vi "Main.vi"() -> ()   [LabVIEW 2017]
uses:
  type defs/action buttons.ctl
  type defs/mode buttons.ctl
  type defs/state.ctl
  type defs/data.ctl
  <vilib>/vision/Image Controls.llb/IMAQ Image.ctl
  type defs/task.ctl
  <vilib>/myRIO/Instrument Drivers/Onboard IO/DIO/typedefs/DIO Reference.ctl
  <vilib>/myRIO/Common/Instrument Driver Framework/Utilities/typedefs/myRIO Generic Hardware Reference.ctl
  <vilib>/myRIO/Common/Instrument Driver Framework/Utilities/typedefs/Hardware Version Enum.ctl
  <vilib>/myRIO/Common/Instrument Driver Framework/Utilities/typedefs/myRIO v1.0 Reference.ctl
  <vilib>/myRIO/Common/Instrument Driver Framework/Utilities/typedefs/Generic FPGA Reference.ctl
  <vilib>/myRIO/Common/Instrument Driver Framework/myRIO v1.0/DIO/typedefs/DIO Channels List.ctl
  <vilib>/myRIO/Common/Instrument Driver Framework/myRIO v1.0/DIO/typedefs/DIO Channels Enum.ctl
  <vilib>/userdefined/High Color/nirio_resource_hc.ctl
  <vilib>/myRIO/Common/Instrument Driver Framework/Utilities/vis/Is FPGA Ref Available.vi
  <vilib>/myRIO/Common/Instrument Driver Framework/myRIO v1.0/DIO/vis/myRIO v1.1 Open DIO.vi
  <vilib>/myRIO/Instrument Drivers/Onboard IO/DIO/vis/Write.vi
  <vilib>/myRIO/Instrument Drivers/Onboard IO/DIO/vis/Read.vi
  <vilib>/myRIO/Common/Instrument Driver Framework/Utilities/vis/Validate Channels.vi
  <vilib>/myRIO/Common/Instrument Driver Framework/myRIO v1.0/DIO/vis/myRIO v1.0 Reserve DIO.vi
  <vilib>/myRIO/Common/Instrument Driver Framework/myRIO v1.0/UART/vis/myRIO v1.0 Close UART.vi
  <vilib>/myRIO/Common/Instrument Driver Framework/myRIO v1.0/Resource Manager/vis/myRIO v1.0 Reserve Channel List.vi
  <vilib>/myRIO/Common/Instrument Driver Framework/myRIO v1.0/DIO/vis/myRIO v1.0 Build MUX Configuration DIO.vi
  <vilib>/myRIO/Common/Instrument Driver Framework/myRIO v1.0/Resource Manager/vis/myRIO v1.0 Reserve Channel.vi
  <vilib>/myRIO/Common/Instrument Driver Framework/myRIO v1.0/Resource Manager/vis/myRIO v1.0 Unreserve Channel.vi
  <vilib>/myRIO/Common/Instrument Driver Framework/myRIO v1.0/Resource Manager/vis/myRIO v1.0 Create Configuration List.vi
  <vilib>/myRIO/Common/Instrument Driver Framework/myRIO v1.0/Resource Manager/vis/myRIO v1.0 Build Mutex Name.vi
  <vilib>/Utility/VariantDataType/GetNumericInfo.vi
  <vilib>/Utility/error.llb/Error Cluster From Error Code.vi
  <vilib>/myRIO/Common/Instrument Driver Framework/myRIO v1.0/myRIO v1.1 Open.vi
  <vilib>/myRIO/Common/Instrument Driver Framework/Utilities/vis/IO Manager.vi
  <vilib>/myRIO/Common/Instrument Driver Framework/Utilities/vis/Configuration Manager.vi
  <vilib>/myRIO/Common/Instrument Driver Framework/myRIO v1.0/Resource Manager/vis/myRIO v1.0 Configure IO.vi
  <vilib>/myRIO/Common/Instrument Driver Framework/myRIO v1.0/myRIO v1.0 Close.vi
  <vilib>/myRIO/Common/Instrument Driver Framework/myRIO v1.0/DIO/vis/myRIO v1.0 Write DIO.vi
  <vilib>/myRIO/Common/Instrument Driver Framework/myRIO v1.0/DIO/vis/myRIO v1.0 Read DIO.vi
  <vilib>/myRIO/Common/Instrument Driver Framework/Utilities/vis/FPGA Ref Manager.vi
  <vilib>/myRIO/Common/Instrument Driver Framework/myRIO v1.0/myRIO v1.0 Reset FPGA.vi
  <vilib>/myRIO/Common/Instrument Driver Framework/myRIO v1.0/IRQ/vis/myRIO v1.0 IRQ Info FGV.vi
  <vilib>/myRIO/Common/Instrument Driver Framework/myRIO v1.0/IRQ/vis/myRIO v1.0 Timer IRQ Info FGV.vi
  <vilib>/myRIO/Common/Instrument Driver Framework/myRIO v1.0/IRQ/vis/myRIO v1.0 ISR Agent.vi
  <vilib>/myRIO/Express VI/Onboard Devices/LED/LED Express VI.xnode
  <vilib>/myRIO/Instrument Drivers/Onboard IO/DIO/vis/myRIO DIO Open.xnode
  <vilib>/myRIO/Express VI/Onboard Devices/Button/Button Express VI.xnode
  <vilib>/vision/NI_Vision_Development_Module.lvlib
  <vilib>/myRIO/Instrument Drivers/Onboard IO/DIO/DIO.lvlib
  <vilib>/myRIO/Instrument Drivers/Utilities/Utilities.lvlib
panel:
  out "error out":errorcluster
  out "Class (Particle Classification 1)":string
  out "number img":i32
  in  "mode buttons":T1
  out "image display":T2(plugin-control)
  in  "action buttons":T3
  in  "Stop":bool
  # "Machine\nVision\nApp"
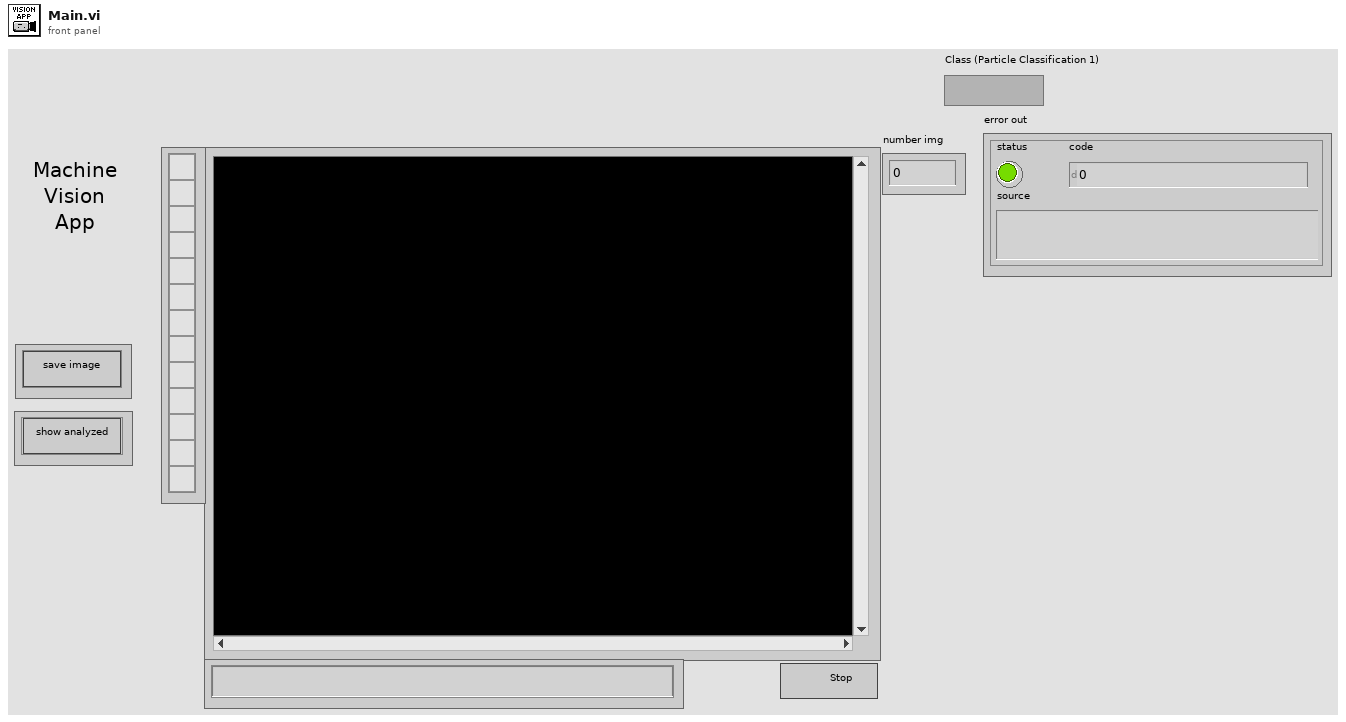
[diagram p1: front panel]
types:
  T1 = typedef "mode buttons.ctl" = cluster{"show analyzed":bool}
  T2 = typedef "IMAQ Image.ctl" = refnum<image>
  T3 = typedef "action buttons.ctl" = cluster{"save image":bool}
  T4 = typedef "data.ctl" = cluster{"save image":bool, "qsm":cluster{"Webcam image ref":T2, "Analyzed image ref":T2, "Stop webcam":bool}, " image ref":T2, "number img":i32}
  T5 = typedef "state.ctl" = enum16{"(qsm) schedule", "(qsm) initialize", "(qsm) release", "(qsm) clean up", "(qsm) shutdown", "(myRIO) initialize", "(myRIO) clean up", "(myRIO) update ports", "(image) get", "(image) analyze", "(image) overlay", "(image) show", "save image", "state A", "state B", "state C", "state D", "state E", "state F", "state G", "state H"}
  T6 = typedef "DIO.lvlib/DIO Reference.ctl" = cluster{"myRIO Reference":T7, "DIO Channels List":T11}
  T7 = typedef "myRIO Generic Hardware Reference.ctl" = cluster{"myRIO Model":T8, "myRIO Hardware Reference":T9}
  T8 = typedef "Hardware Version Enum.ctl" = enum16{"Unknown", "myRIO-1900", "myRIO-1950", "roboRIO", "NI ELVIS RIO CM"}
  T9 = typedef "myRIO v1.0 Reference.ctl" = cluster{"Generic FPGA Reference":T10, "Allow multiple opens":bool}
  T10 = typedef "Generic FPGA Reference.ctl" = refnum<k20>
  T11 = typedef "DIO Channels List.ctl" = T12[]
  T12 = typedef "DIO Channels Enum.ctl" = enum16{"Not Connected", "C/DIO0", "C/DIO1", "C/DIO2", "C/DIO3", "C/DIO4", "C/DIO5", "C/DIO6", "C/DIO7", "A/DIO0", "A/DIO1", "A/DIO2", "A/DIO3", "A/DIO4", "A/DIO5", "A/DIO6", "A/DIO7", "A/DIO8", "A/DIO9", "A/DIO10", "A/DIO11", "A/DIO12", "A/DIO13", "A/DIO14", "A/DIO15", "B/DIO0", "B/DIO1", "B/DIO2", "B/DIO3", "B/DIO4", "B/DIO5", "B/DIO6", "B/DIO7", "B/DIO8", "B/DIO9", "B/DIO10", "B/DIO11", "B/DIO12", "B/DIO13", "B/DIO14", "B/DIO15", "LED0", "LED1", "LED2", "LED3", "Button0", "DIO/DIO0", "DIO/DIO1", "DIO/DIO2", "DIO/DIO3", "DIO/DIO4", "DIO/DIO5", "DIO/DIO6", "DIO/DIO7", "DIO/DIO8", "DIO/DIO9", "SPI/CS0", "SPI/CS1", "SPI/CS2", "SPI/CS3", "LED RADIO (Green)", "LED RADIO (Red)", "LED COMM (Green)", "LED COMM (Red)", "LED MODE (Green)", "LED MODE (Red)"}
  T13 = typedef "nirio_resource_hc.ctl" = tag
  T14 = typedef "task.ctl" = T5[]
  T15 = typedef "Image Type" = u32
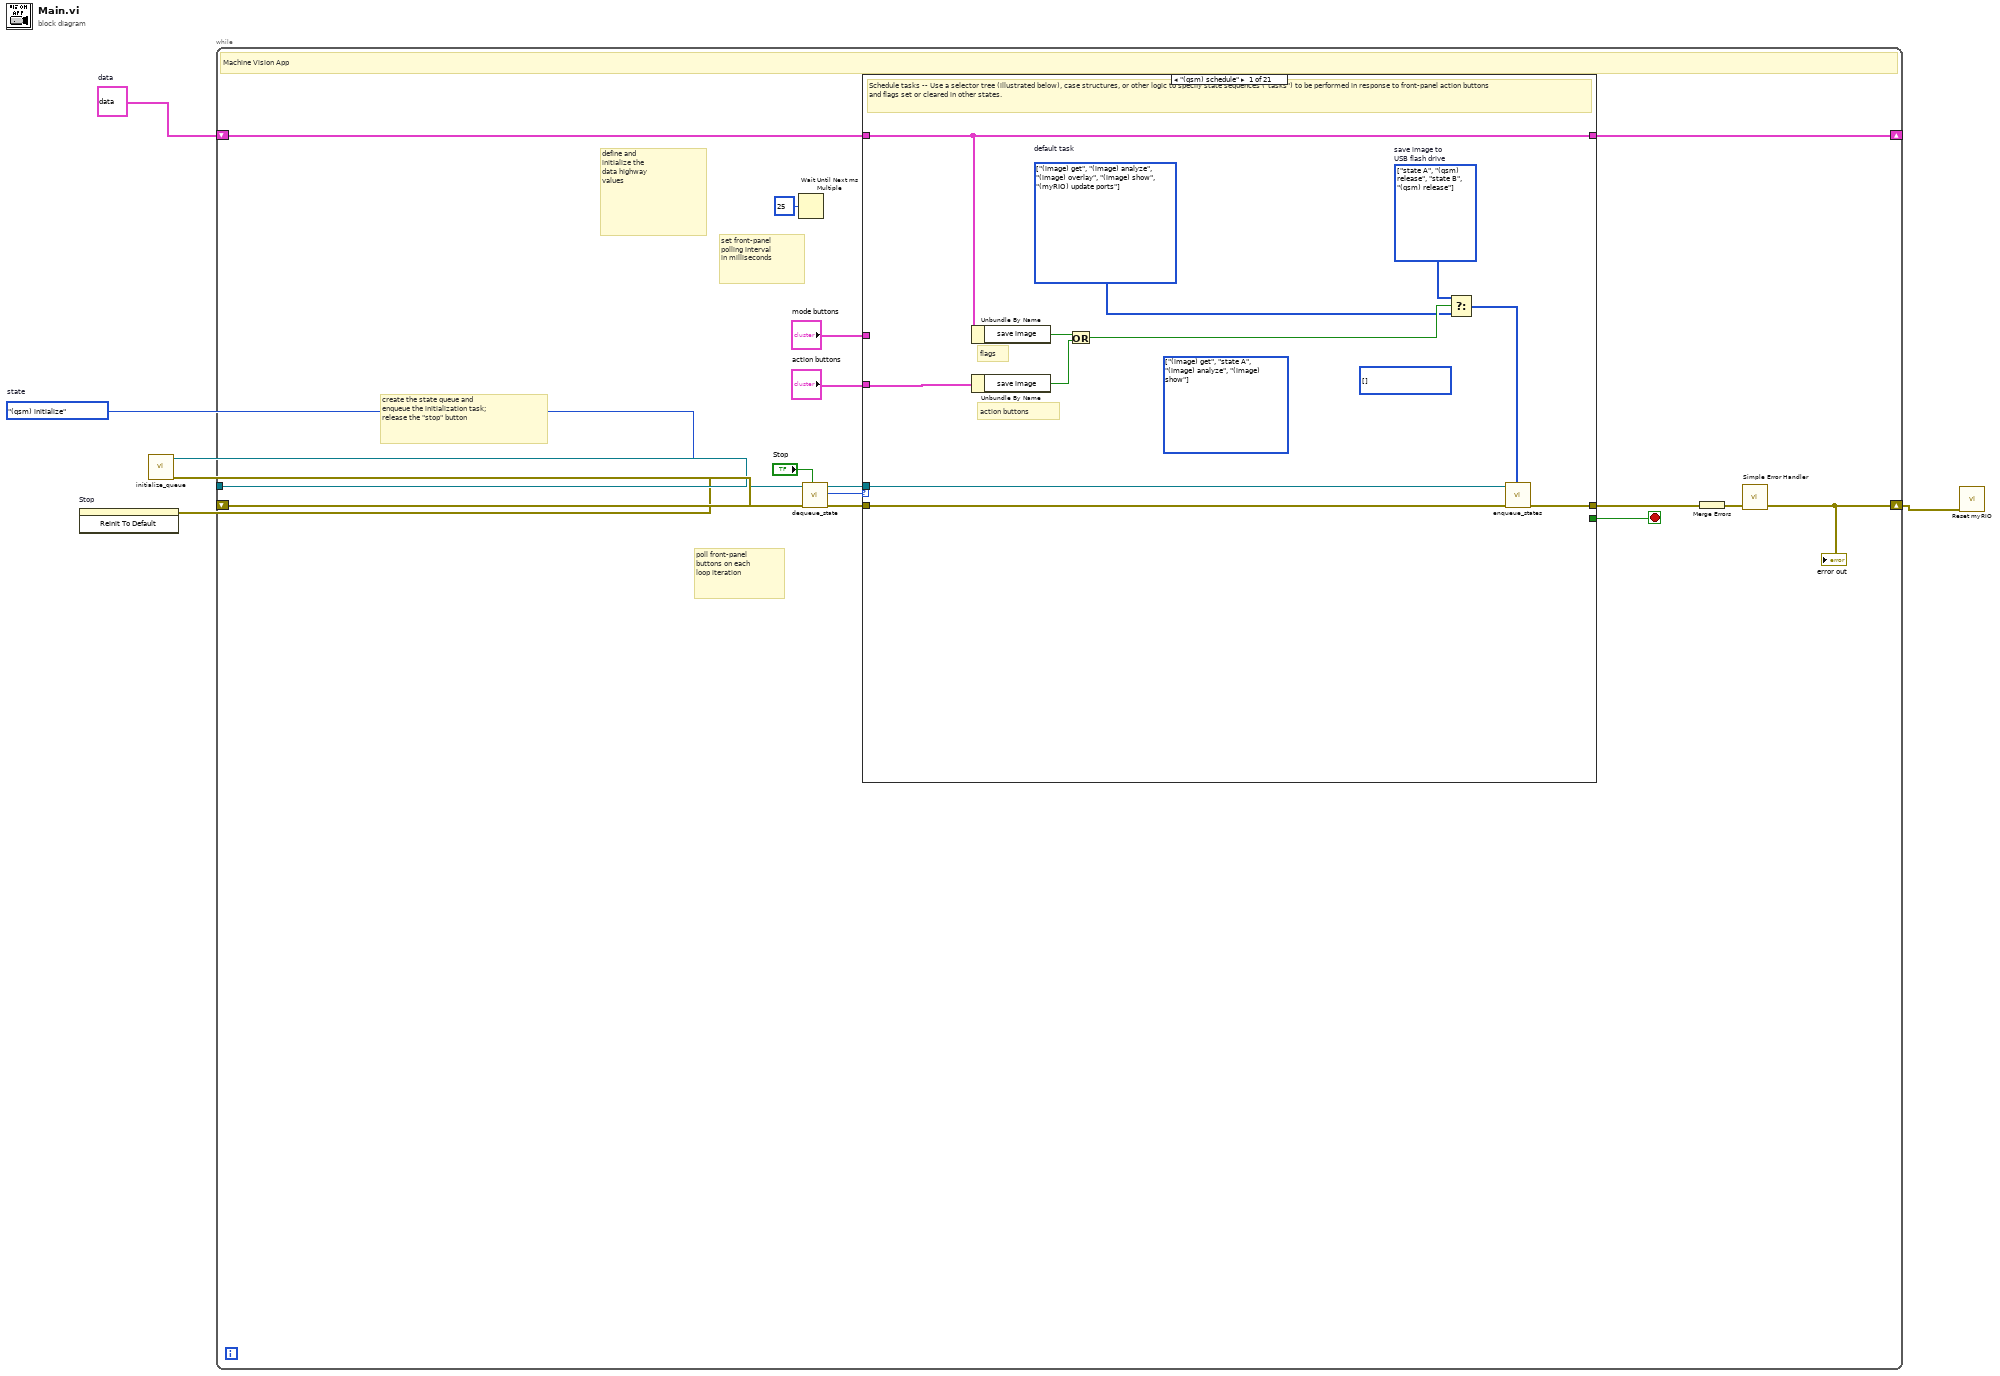
[diagram p0: block diagram]
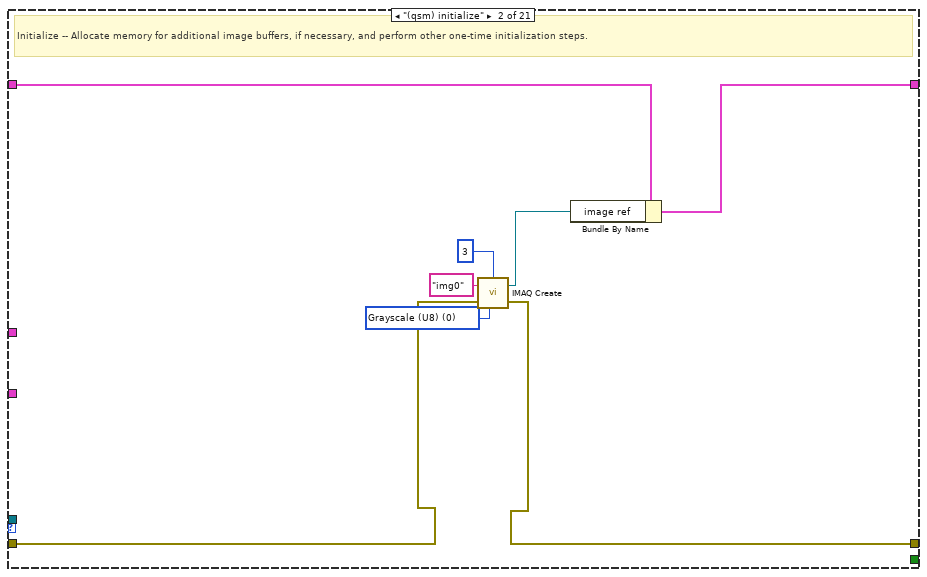
[diagram p2: hidden frame]
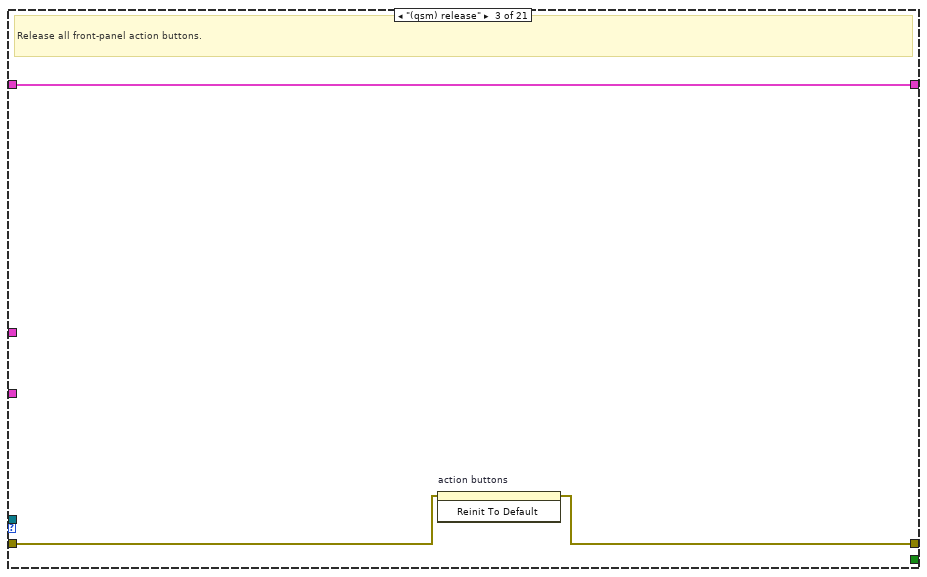
[diagram p3: hidden frame]
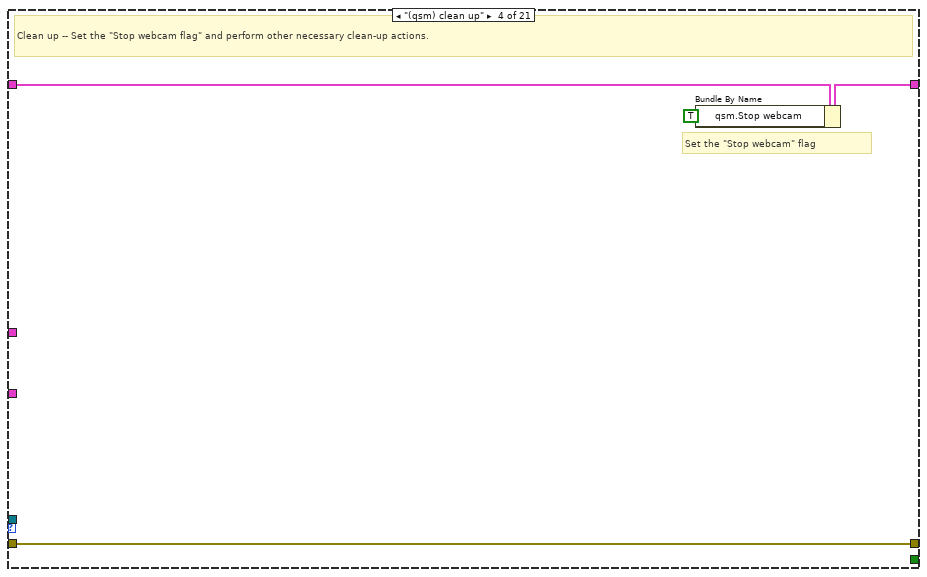
[diagram p4: hidden frame]
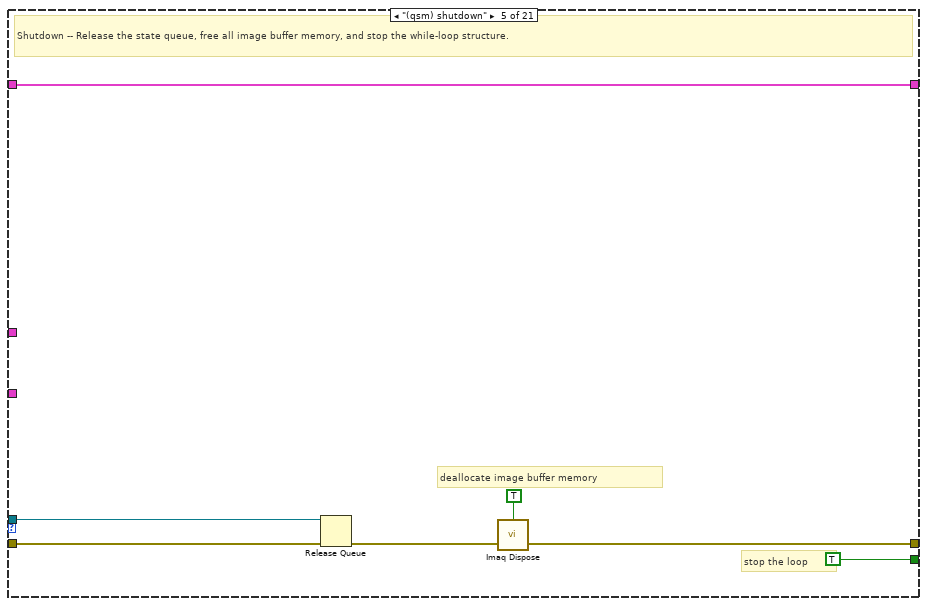
[diagram p5: hidden frame]
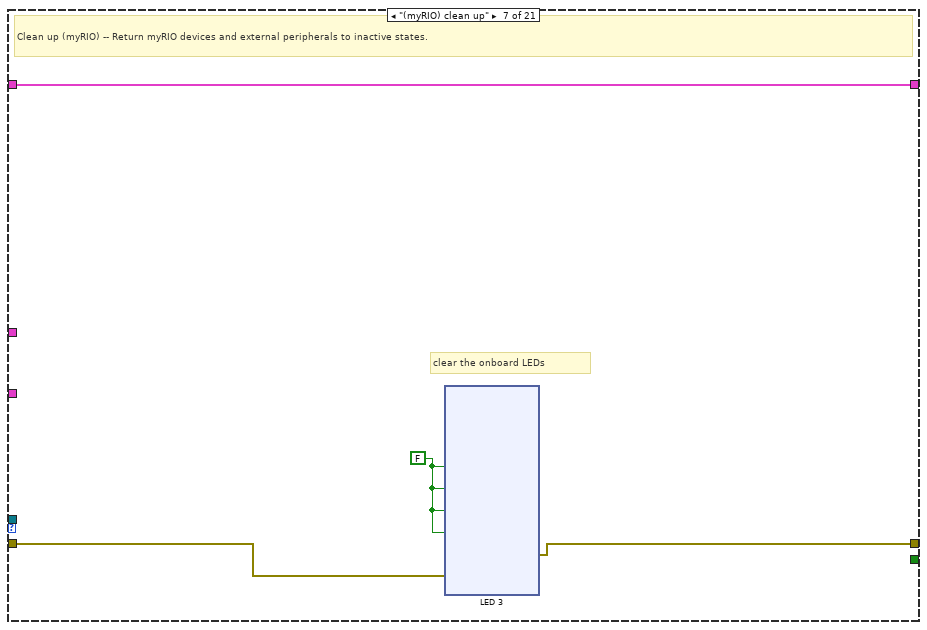
[diagram p7: hidden frame]
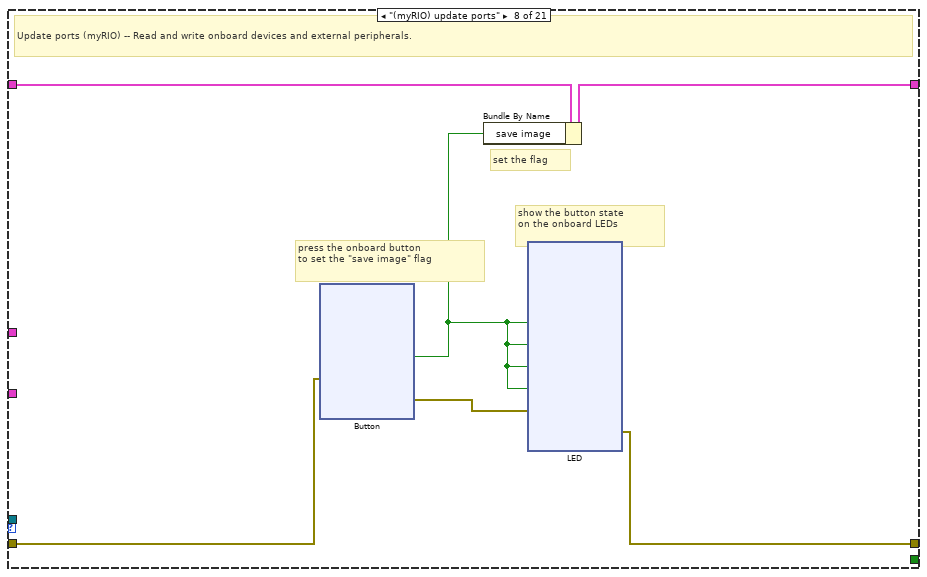
[diagram p8: hidden frame]
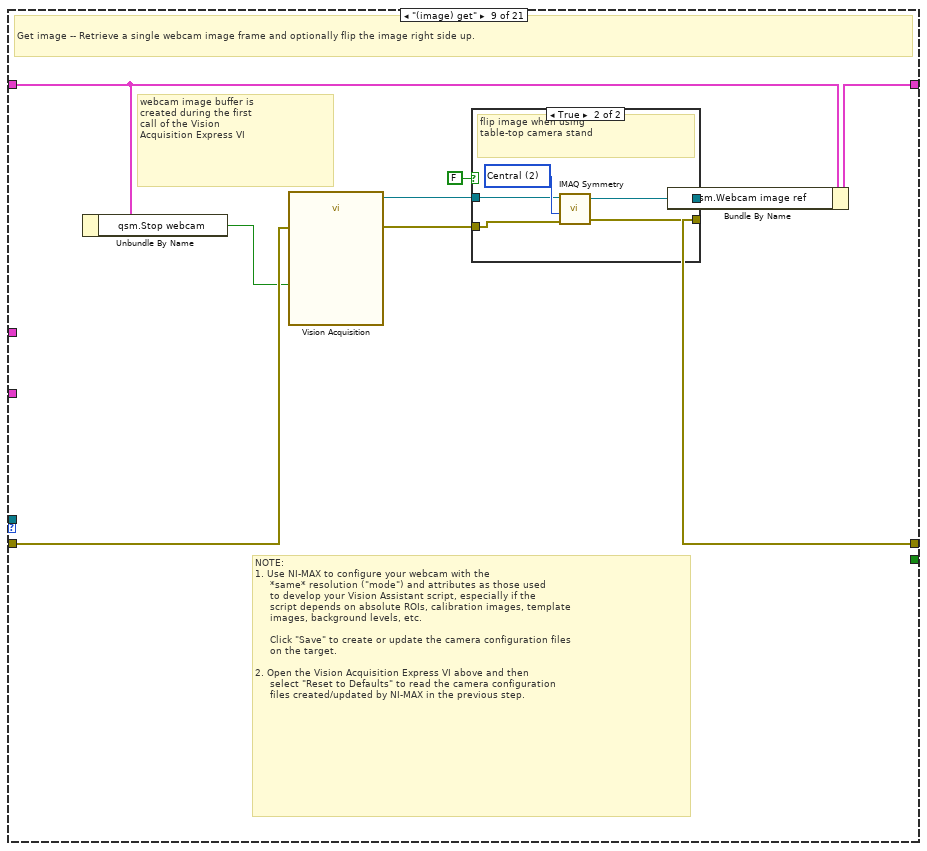
[diagram p9: hidden frame]
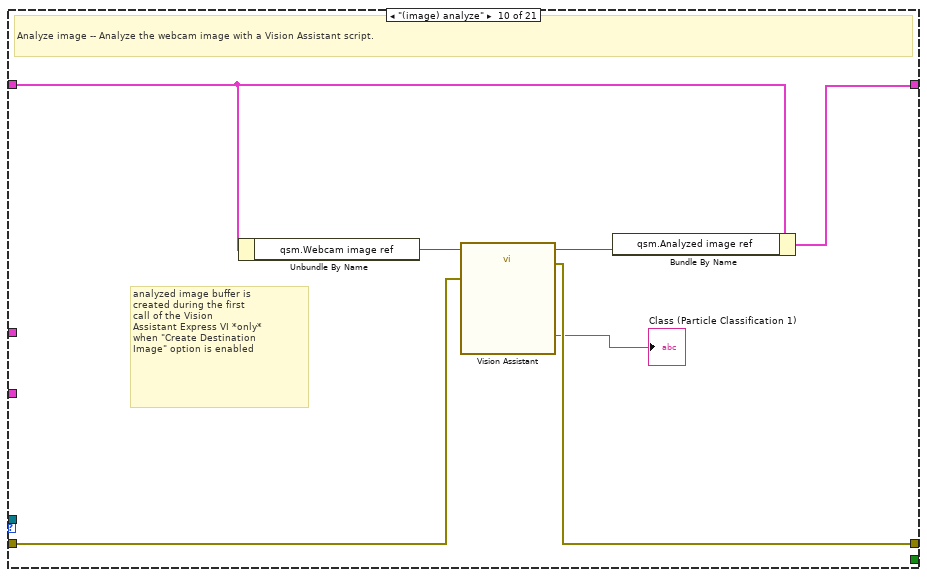
[diagram p11: hidden frame]
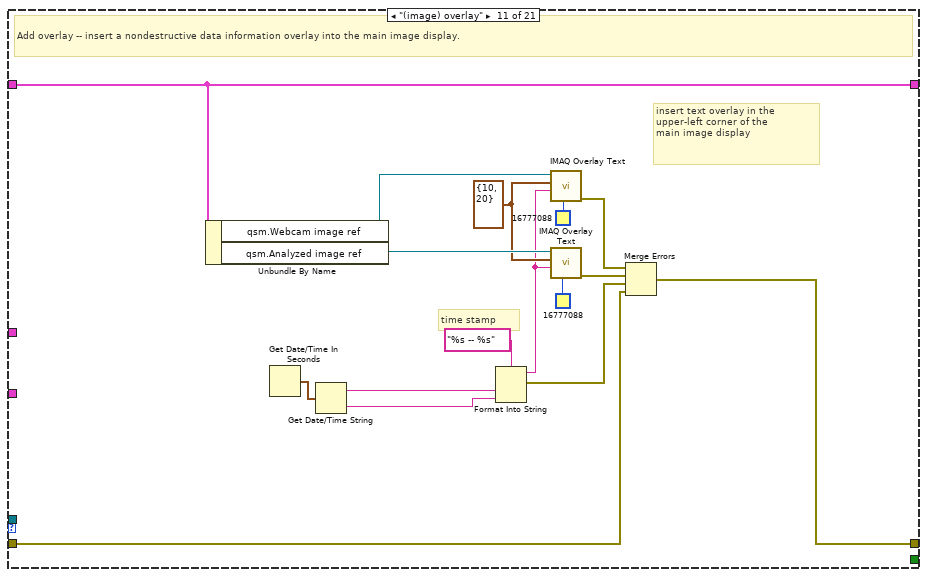
[diagram p12: hidden frame]
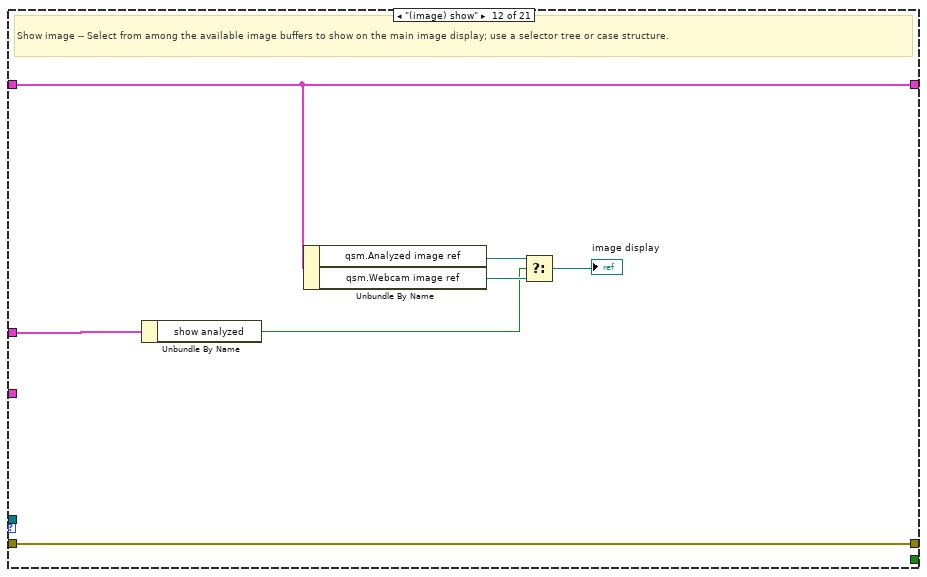
[diagram p13: hidden frame]
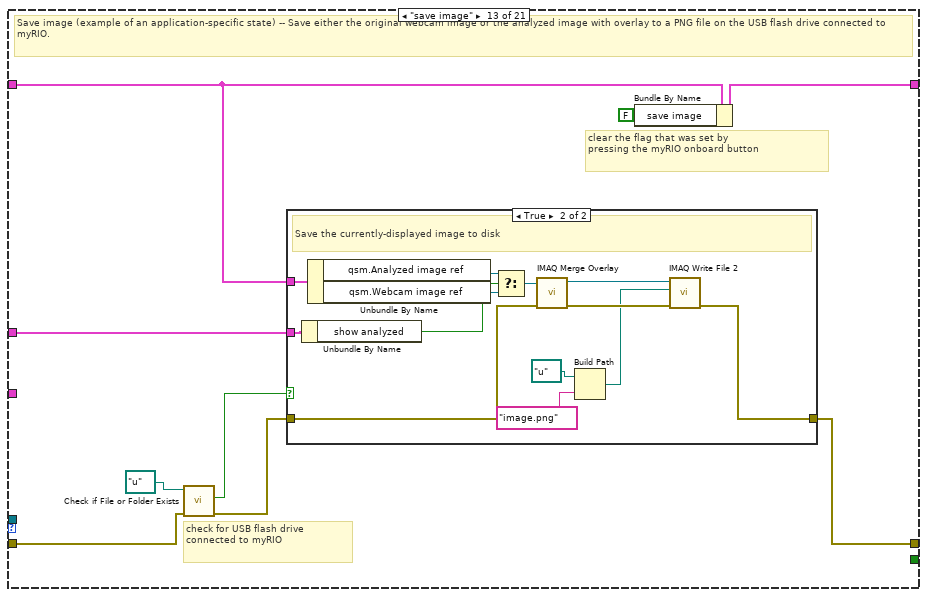
[diagram p14: hidden frame]
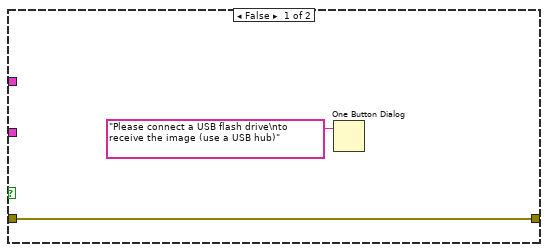
[diagram p15: hidden frame]
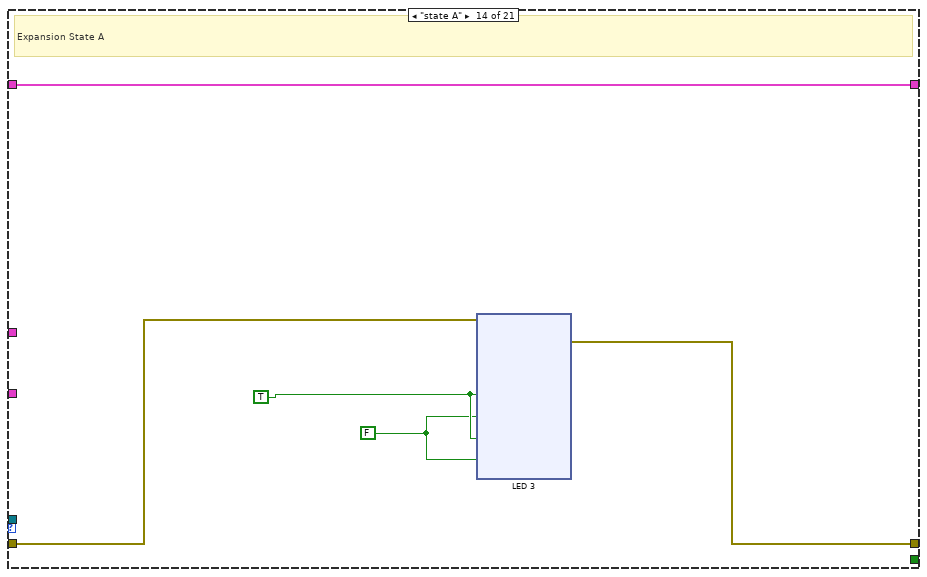
[diagram p16: hidden frame]
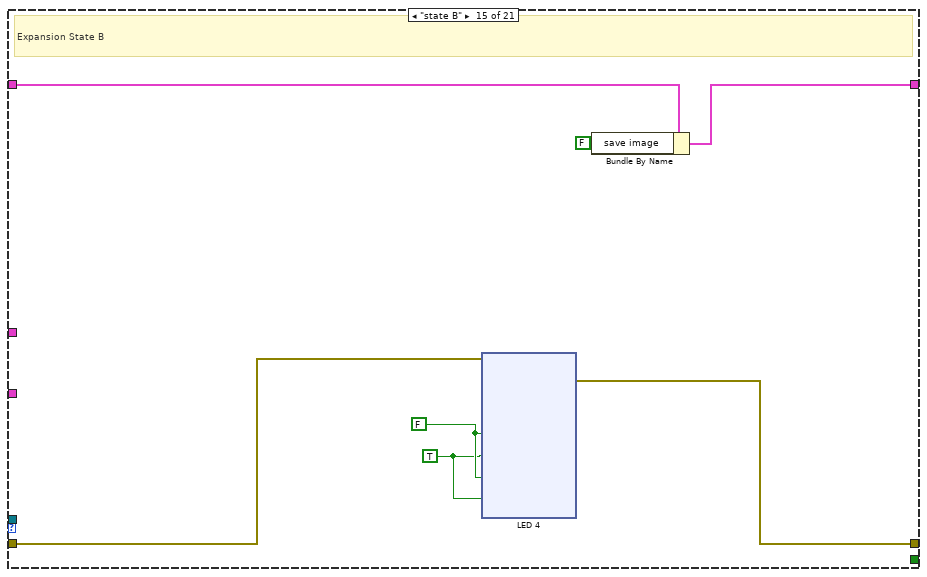
[diagram p17: hidden frame]
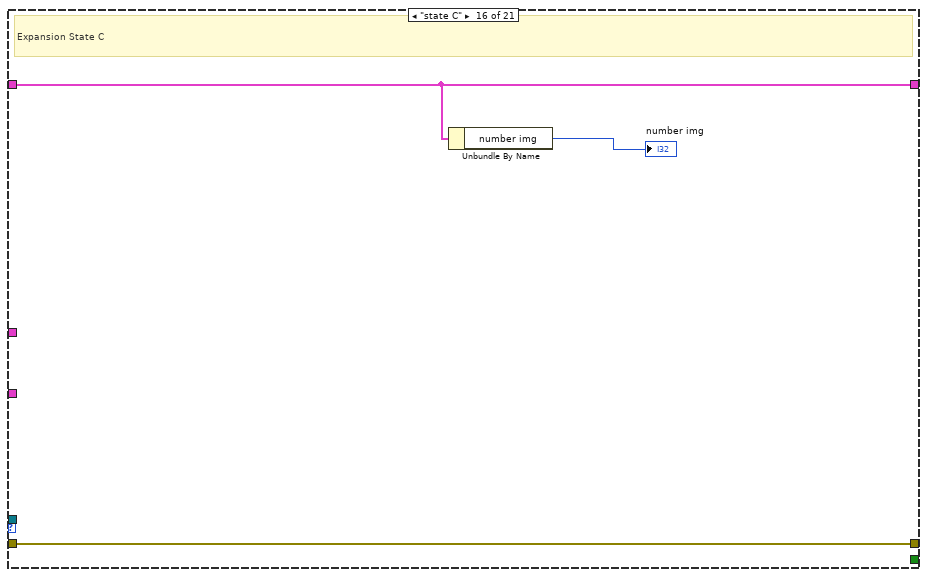
[diagram p18: hidden frame]
diagram:
  w6 = T4 {"save image"=FALSE, "qsm"={"Webcam image ref"=refnum, "Analyzed image ref"=refnum, "Stop webcam"=FALSE}, " image ref"=refnum, "number img"=0}  # data
  w2 = state."(qsm) initialize"  # state
  n1 = invoke on="Stop" class="Bool" method="Reinit To Default"() -> (error out=w3:errorcluster)  [unwired: 3 in, 2 out]
  n2 = call "initialize_queue.vi"("error in (no error)"=w3, "state"=w2) -> ("error out"=w5:errorcluster, "queue out"=w4:refnum<queue>)  [unwired: 8 in]
  n3 = while {
    shift-right: [w7] -> w1
    shift-left: w5 -> [w13]
    tunnel: w4 -> [w14]
    shift-right: [w17] -> _
    shift-left: w6 -> [w18]
    stop <- w16 stop-if-true
    # "define and \ninitialize the \ndata highway\nvalues"
    # "create the state queue and\nenqueue the initialization task;\nrelease the \"stop\" button"
    # "set front-panel\npolling interval\nin milliseconds"
    # "poll front-panel\nbuttons on each\nloop iteration"
    # "Machine Vision App"
    n4 = Wait Until Next ms Multiple(millisecond multiple=u32 25) -> ()  [unwired: 1 out]
    n5 = call "dequeue_state.vi"("stop"="Stop", "error in (no error)"=w13, "queue in"=w14) -> ("error out"=w15:errorcluster, "state"=w8:T5, "queue out"=w11:refnum<queue>)  [unwired: 6 in]
    n6 = case shown="\"(qsm) schedule\"" w8 {
      tunnel: w15 -> [w27 w39 w41 w43 w52 w54 w57 w101 w185 w195 w200 w218 w226 w250 w293 w337 w339 w341 w342 w344 w347]
      tunnel: w11 -> [w28 _ _ _ w51 _ _ _ _ _ _ _ _ _ _ _ _ _ _ _ _]
      tunnel: [w29 w38 w40 w43 w47 w54 w56 w99 w180 w194 w209 w218 w227 w247 w294 w337 w339 w341 w342 w344 w347] -> w20
      tunnel: "action buttons" -> [w31 _ _ _ _ _ _ _ _ _ _ _ _ _ _ _ _ _ _ _ _]
      tunnel: w18 -> [w30 w33 w42 w45 w50 w55 w59 w103 w178 w199 w201 w219 w231 w251 w292 w336 w338 w340 w343 w345 w346]
      tunnel: [w30 w32 w42 w44 w50 w55 w59 w102 w184 w198 w201 w219 w230 w251 w290 w336 w338 w340 w343 w345 w346] -> w17
      tunnel: [_ _ _ _ TRUE _ _ _ _ _ _ _ _ _ _ _ _ _ _ _ _] -> w16
      tunnel: "mode buttons" -> [_ _ _ _ _ _ _ _ _ _ _ w217 w228 _ _ _ _ _ _ _ _]
      frame "(qsm) schedule" {
        (unwired) T14 [enum."(image) get", enum."state A", enum."(image) analyze", enum."(image) show"] items=["(qsm) schedule", "(qsm) initialize", "(qsm) release", "(qsm) clean up", "(qsm) shutdown", "(myRIO) initialize", "(myRIO) clean up", "(myRIO) update ports", "(image) get", "(image) analyze", "(image) overlay", "(image) show", "save image", "state A", "state B", "state C", "state D", "state E", "state F", "state G", "state H"] ("task")
        (unwired) T5[] [] items=["(qsm) schedule", "(qsm) initialize", "(qsm) release", "(qsm) clean up", "(qsm) shutdown", "(myRIO) initialize", "(myRIO) clean up", "(myRIO) update ports", "(image) get", "(image) analyze", "(image) overlay", "(image) show", "save image", "state A", "state B", "state C", "state D", "state E", "state F", "state G", "state H"]
        w23 = T14 [enum."state A", enum."(qsm) release", enum."state B", enum."(qsm) release"] items=["(qsm) schedule", "(qsm) initialize", "(qsm) release", "(qsm) clean up", "(qsm) shutdown", "(myRIO) initialize", "(myRIO) clean up", "(myRIO) update ports", "(image) get", "(image) analyze", "(image) overlay", "(image) show", "save image", "state A", "state B", "state C", "state D", "state E", "state F", "state G", "state H"]  # save image to USB flash drive
        w21 = T14 [enum."(image) get", enum."(image) analyze", enum."(image) overlay", enum."(image) show", enum."(myRIO) update ports"] items=["(qsm) schedule", "(qsm) initialize", "(qsm) release", "(qsm) clean up", "(qsm) shutdown", "(myRIO) initialize", "(myRIO) clean up", "(myRIO) update ports", "(image) get", "(image) analyze", "(image) overlay", "(image) show", "save image", "state A", "state B", "state C", "state D", "state E", "state F", "state G", "state H"]  # default task
        # "action buttons"
        # "flags"
        # "Schedule tasks -- Use a selector tree (illustrated below), case structures, or other logic to specify state sequences (\"tasks\") to be performed in response to front-panel action buttons and flags set or cleared in other states."
        n7 = Unbundle By Name "Unbundle By Name"(w30) -> ("save image"=w26:bool)
        n8 = Unbundle By Name(w31) -> ("save image"=w25:bool)
        n9 = Or(x=w26, y=w25) -> (x .or. y?=w24:bool)
        n10 = Select(t=w23, s=w24, f=w21) -> (s? t:f=w22:T14)
        n11 = call "enqueue_states.vi"("task"=w22, "error in"=w27, "queue in"=w28) -> ("error out"=w29:errorcluster)  [unwired: 6 in, 1 out]
      }
      frame "(qsm) initialize" {
        w36 = T15 0 items=["Grayscale (U8)", "Grayscale (I16)", "Grayscale (SGL)", "Complex (CSG)", "RGB (U32)", "HSL (U32)", "RGB (U64)", "Grayscale (U16)"] ("Image Type")
        # "Initialize -- Allocate memory for additional image buffers, if necessary, and perform other one-time initialization steps."
        n12 = call "IMAQ Create"("Border Size"=3, "Image Name"="img0", "Image Type"=w36, "error in (no error)"=w39) -> ("New Image"=w34:T2, "error out"=w38:errorcluster)  [unwired: 1 in]
        n13 = Bundle By Name(cluster=w33, "image ref"=w34) -> (w32:T4)
      }
      frame "(qsm) release" {
        # "Release all front-panel action buttons."
        n14 = invoke on="action buttons" class="Clust (strict)" method="Reinit To Default"(error in=w41) -> (error out=w40:errorcluster)  [unwired: 2 in, 2 out]
      }
      frame "(qsm) clean up" {
        # "Set the \"Stop webcam\" flag"
        # "Clean up -- Set the \"Stop webcam flag\" and perform other necessary clean-up actions."
        n15 = Bundle By Name(cluster=w45, "qsm.Stop webcam"=TRUE) -> (w44:T4)
      }
      frame "(qsm) shutdown" {
        # "deallocate image buffer memory"
        # "stop the loop"
        # "Shutdown -- Release the state queue, free all image buffer memory, and stop the while-loop structure."
        n16 = Release Queue(queue=w51, error in (no error)=w52) -> (error out=w48:errorcluster)  [unwired: 1 in, 2 out]
        n17 = call "Imaq Dispose"("All Images? (No)"=TRUE, "error in (no error)"=w48) -> ("error out"=w47:errorcluster)  [unwired: 4 in]
      }
      frame "(myRIO) initialize" {
        # "Initialize (myRIO) -- Open channels, configure devices, send setup strings to peripherals, etc."
      }
      frame "(myRIO) clean up" {
        w58 = FALSE ("LED3")
        # "clear the onboard LEDs"
        # "Clean up (myRIO) -- Return myRIO devices and external peripherals to inactive states."
        n18 = xnode "LED 3"("LED0"=w58, "LED1"=w58, "LED2"=w58, "LED3"=w58, "error in (no error)"=w57) -> ("error out"=w56:errorcluster)
      }
      frame "(myRIO) update ports" {
        # "show the button state\non the onboard LEDs"
        # "set the flag"
        # "press the onboard button\nto set the \"save image\" flag"
        # "Update ports (myRIO) -- Read and write onboard devices and external peripherals."
        n19 = xnode "Button"("error in (no error)"=w101) -> ("Value"=w98:bool, "error out"=w100:errorcluster)
        n20 = Bundle By Name "Bundle By Name"(cluster=w103, "save image"=w98) -> (w102:T4)
        n21 = xnode "LED"("LED0"=w98, "LED1"=w98, "LED2"=w98, "LED3"=w98, "error in (no error)"=w100) -> ("error out"=w99:errorcluster)
      }
      frame "(image) get" {
        # "webcam image buffer is\ncreated during the first\ncall of the Vision\nAcquisition Express VI"
        # "NOTE:\n1. Use NI-MAX to configure your webcam with the\n     *same* resolution (\"mode\") and attributes as those used \n     to develop your Vision Assistant script, especially if the\n     script depends on absolute ROIs, calibration images, template\n     images, background levels, etc.\n \n     Click \"Save\" to create or update the camera configuration files\n     on the target.\n\n2. Open the Vision Acquisition Express VI above and then\n     select \"Reset to Defaults\" to read the camera configuration\n     files created/updated by NI-MAX in the previous step."
        # "Get image -- Retrieve a single webcam image frame and optionally flip the image right side up."
        n22 = Unbundle By Name(w178) -> ("qsm.Stop webcam"=w177:bool)
        n23 = call "Vision Acquisition"("Stop (F)"=w177, "error in"=w185) -> ("Image Out"=w183:T2, "error out"=w181:errorcluster)  [unwired: 23 in, 1 out]
        n24 = case shown="True" FALSE {
          tunnel: w183 -> [w187 w191]
          tunnel: [w187 w190] -> w182
          tunnel: w181 -> [w186 w189]
          tunnel: [w186 w188] -> w180
          frame False {
            # "use webcam image as-is"
          }
          frame True {
            w192 = u32 2 items=["Horizontal", "Vertical", "Central", "1st Diagonal", "2nd Diagonal"] ("Type of Symmetry")
            # "flip image when using\ntable-top camera stand"
            n25 = call "IMAQ Symmetry"("error in (no error)"=w189, "Type of Symmetry"=w192, "Image Src"=w191) -> ("error out"=w188:errorcluster, "Image Dst Out"=w190:T2)  [unwired: 2 in]
          }
        }
        n26 = Bundle By Name(cluster=w178, "qsm.Webcam image ref"=w182) -> (w184:T4)
      }
      frame "(image) analyze" {
        # "analyzed image buffer is\ncreated during the first\ncall of the Vision\nAssistant Express VI *only*\nwhen \"Create Destination\nImage\" option is enabled"
        # "Analyze image -- Analyze the webcam image with a Vision Assistant script."
        n27 = Unbundle By Name "Unbundle By Name"(w199) -> ("qsm.Webcam image ref"=w197:T2)
        n28 = call "Vision Assistant"("Image In"=w197, "error in"=w195) -> ("Image Out"=w196:T2, "error out"=w194:errorcluster, "Class (Particle Classification 1)"=→"Class (Particle Classification 1)":string)  [unwired: 23 in]
        n29 = Bundle By Name "Bundle By Name"(cluster=w199, "qsm.Analyzed image ref"=w196) -> (w198:T4)
      }
      frame "(image) overlay" {
        w211 = cluster{"X":i32, "Y":i32} {"X"=10, "Y"=20} ("Origin")
        # "time stamp"
        # "insert text overlay in the\nupper-left corner of the \nmain image display"
        # "Add overlay -- insert a nondestructive data information overlay into the main image display."
        n30 = Unbundle By Name "Unbundle By Name"(w201) -> ("qsm.Webcam image ref"=w212:T2, "qsm.Analyzed image ref"=w215:T2)
        n31 = Get Date/Time In Seconds() -> (seconds since 1Jan1904=w205:timestamp)
        n32 = Get Date/Time String(seconds (now)=w205) -> (date string=w204:string, time string=w203:string)  [unwired: 2 in]
        n33 = Format Into String "Format Into String"(format string="%s -- %s", w204, w203) -> (resulting string=w206:string, error out=w202:errorcluster)  [unwired: 2 in]
        n34 = call "IMAQ Overlay Text"("Text Color (black)"=u32 16777088, "String"=w206, "Origin"=w211, "Image"=w212) -> ("error out"=w208:errorcluster)  [unwired: 6 in, 1 out]
        n35 = call "IMAQ Overlay Text"("Text Color (black)"=u32 16777088, "String"=w206, "Origin"=w211, "Image"=w215) -> ("error out"=w210:errorcluster)  [unwired: 6 in, 1 out]
        n36 = Merge Errors "Merge Errors"(w208, w210, w202, w200) -> (w209:errorcluster)
      }
      frame "(image) show" {
        # "Show image -- Select from among the available image buffers to show on the main image display; use a selector tree or case structure."
        n37 = Unbundle By Name "Unbundle By Name"(w217) -> ("show analyzed"=w216:bool)
        n38 = Unbundle By Name "Unbundle By Name"(w219) -> ("qsm.Analyzed image ref"=w222:T2, "qsm.Webcam image ref"=w221:T2)
        n39 = Select(t=w222, s=w216, f=w221) -> (s? t:f=→"image display":T2)
      }
      frame "save image" {
        # "check for USB flash drive\nconnected to myRIO"
        # "clear the flag that was set by\npressing the myRIO onboard button"
        # "Save image (example of an application-specific state) -- Save either the original webcam image or the analyzed image with overlay to a PNG file on the USB flash drive connected to myRIO."
        n40 = call <vilib>:"Check if File or Folder Exists.vi"("error in (no error)"=w226, "path"=path "u:/") -> ("error out"=w225:errorcluster, "file or folder exists?"=w224:bool)  [unwired: 7 in, 1 out]
        n41 = case shown="True" w224 {
          tunnel: w231 -> [_ w244]
          tunnel: w228 -> [_ w243]
          tunnel: [w232 w242] -> w227
          tunnel: w225 -> [w232 w240]
          frame False {
            n42 = One Button Dialog(message="Please connect a USB flash drive\nto receive the image (use a USB hub)") -> ()  [unwired: 1 in, 1 out]
          }
          frame True {
            # "Save the currently-displayed image to disk"
            n43 = Unbundle By Name(w243) -> ("show analyzed"=w241:bool)
            n44 = Unbundle By Name(w244) -> ("qsm.Analyzed image ref"=w239:T2, "qsm.Webcam image ref"=w245:T2)
            n45 = Select(t=w239, s=w241, f=w245) -> (s? t:f=w238:T2)
            n46 = call "IMAQ Merge Overlay"("error in (no error)"=w240, "Image Src"=w238) -> ("error out"=w246:errorcluster, "Image Dst Out"=w237:T2)  [unwired: 8 in]
            n47 = Build Path(base path=path "u:/", name or relative path="image.png") -> (appended path=w235:path)
            n48 = call-poly "IMAQ Write File 2"("error in (no error)"=w246, "File Path"=w235, "Image"=w237) -> ("error out"=w242:errorcluster)  [unwired: 7 in, 1 out]
          }
        }
        n49 = Bundle By Name(cluster=w231, "save image"=FALSE) -> (w230:T4)
      }
      frame "state A" {
        w248 = FALSE
        w249 = TRUE
        # "Expansion State A"
        n50 = xnode "LED 3"("LED0"=w249, "LED1"=w248, "LED2"=w249, "LED3"=w248, "error in (no error)"=w250) -> ("error out"=w247:errorcluster)
      }
      frame "state B" {
        w295 = TRUE ("LED1")
        w296 = FALSE ("LED0")
        # "Expansion State B"
        n51 = xnode "LED 4"("LED0"=w296, "LED1"=w295, "LED2"=w296, "LED3"=w295, "error in (no error)"=w293) -> ("error out"=w294:errorcluster)
        n52 = Bundle By Name(cluster=w292, "save image"=FALSE) -> (w290:T4)
      }
      frame "state C" {
        # "Expansion State C"
        n53 = Unbundle By Name(w336) -> ("number img"=→"number img":i32)
      }
      frame "state D" {
        # "Expansion State D"
      }
      frame "state E" {
        # "Expansion State E"
      }
      frame "state F" {
        # "Expansion State F"
      }
      frame "state G" {
        # "Expansion State G"
      }
      frame "state H" {
        # "Expansion State H"
      }
    }
    n54 = Merge Errors(w20) -> (w7:errorcluster)
    "error out" <- w7
    n55 = call <vilib>:"Simple Error Handler.vi"() -> ()  [unwired: 5 in, 5 out]
  }
  n56 = call <vilib>:"Reset myRIO.vi"("error in (no error)"=w1) -> ()  [unwired: 10 in, 1 out]
